vi "Release.vi"(8 "Error In":errorcluster, 11 "String In":refnum<class "String.lvclass">) -> (0 "Error Out":errorcluster)   [LabVIEW 2016, in "String.lvclass"]
uses:
  String.lvclass
  Tree Data/Tree Data.lvclass
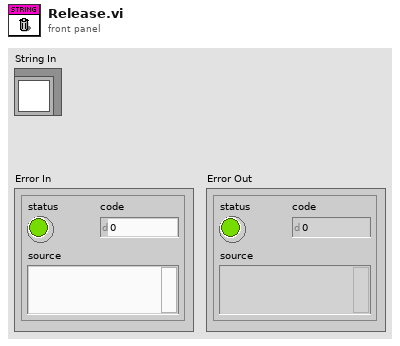
[diagram p1: front panel]
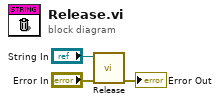
[diagram p0: block diagram]
diagram:
  n1 = call-parent "Release.vi"("Error In"="Error In", "Tree Data In"="String In") -> ("Error Out"=→"Error Out":errorcluster)  [unwired: 9 in]
